vi "Kalman_Filter_Update.vi"(8 "error in":errorcluster, 9 "T Sample":dbl, 10 "New Measurement":dbl, 11 "Kalman_Filter in":refnum<class "Kalman_Filter.lvclass">) -> (0 "error out":errorcluster, 2 "Estimate":dbl, 3 "Kalman_Filter out":refnum<class "Kalman_Filter.lvclass">)   [LabVIEW 2021, in "Kalman_Filter.lvclass"]
uses:
  Kalman_Filter.lvclass
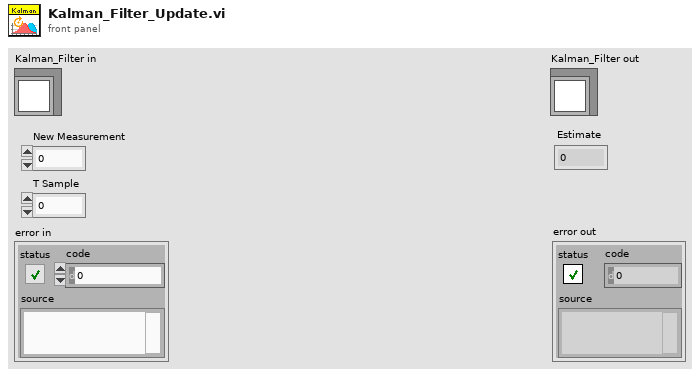
[diagram p1: front panel]
types:
  T1 = cluster{"State":dbl[][], "F state prop matrix":dbl[][], "H measure matrix":dbl[][], "P process cov":dbl[][], "R measure cov":dbl[][], "Q state cov":dbl[][], "T Sample":dbl, "New Measurement":dbl, "Measurement Variance":dbl, "State Variance":dbl, "Threshold":dbl, "Initialized":bool}
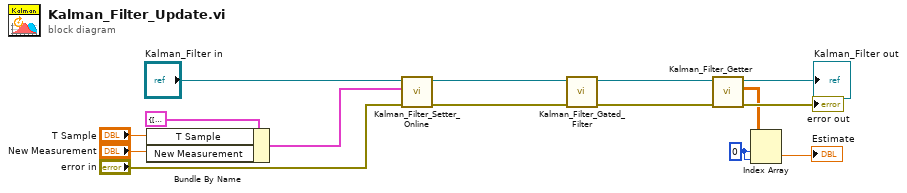
[diagram p0: block diagram]
diagram:
  w2 = 0 ("index (row)")
  n1 = Bundle By Name(cluster=T1 {"State"=[], "F state prop matrix"=[], "H measure matrix"=[], "P process cov"=[], "R measure cov"=[], "Q state cov"=[], "T Sample"=0.0, "New Measurement"=0.0, "Measurement Variance"=0.0, "State Variance"=0.0, "Threshold"=0.0, "Initialized"=FALSE} ("KF"), "T Sample"="T Sample", "New Measurement"="New Measurement") -> (w9:T1)
  n2 = call-dynamic "Kalman_Filter_Setter_Online.vi"("error in (no error)"="error in", "KF"=w9, "Kalman_Filter in"="Kalman_Filter in") -> ("error out"=w7:errorcluster, "Kalman_Filter out"=w6:refnum<class "Kalman_Filter.lvclass">)  [unwired: 7 in]
  n3 = call-dynamic "Kalman_Filter_Gated_Filter.vi"("error in (no error)"=w7, "Kalman_Filter in"=w6) -> ("error out"=w12:errorcluster, "Kalman_Filter out"=w13:refnum<class "Kalman_Filter.lvclass">)  [unwired: 8 in]
  n4 = call-dynamic "Kalman_Filter_Getter.vi"("error in (no error)"=w12, "Kalman_Filter in"=w13) -> ("error out"=→"error out":errorcluster, "State"=w3:dbl[][], "Kalman_Filter out"=→"Kalman_Filter out":refnum<class "Kalman_Filter.lvclass">)  [unwired: 6 in, 1 out]
  n5 = Index Array(array=w3, index (row)=w2, index (col)=w2) -> (element=→"Estimate":dbl)
